vi "ZLIB Transfer Raw File__ogtk.vi"(5 "error in (no error)":errorcluster, 6 "compressed size":u32, 7 "unzip Refnum":T1, 8 "zip Refnum":T2) -> (0 "error out":errorcluster, 2 "unzip Refnum out":T1, 3 "zip Refnum out":T2)   [LabVIEW 2012]
doc: "Copies a file in raw mode from an unzip session into the ZIP file. Both file sessions must have been opened in raw mode, otherwise the created archive will be corrupted."
uses:
  <userlib>/_OpenG.lib/lvzip/lvzip.llb/ZLIB Unzip Handle__ogtk.ctl
  <userlib>/_OpenG.lib/lvzip/lvzip.llb/ZLIB Zip Handle__ogtk.ctl
  <userlib>/_OpenG.lib/lvzip/lvzlib.dll
panel:
  # "Please visit http://www.OpenG.org to learn about the\nOpen Source LabVIEW software movement.\n\nNOTICE -- YOU MUST LEAVE THIS NOTICE IN PLACE.  PER THE TERMS OF THE LICENSE BELOW, YOU MAY SUBLICENSE THIS SOFTWARE \nIN ANY WAY THAT DOES NOT CONFLICT WITH THIS LICENSE.\n\n### BSD License (http://www.opensource.org/licenses/bsd-license.php) Begin ###\n \nCopyright (C) 2002-2004 Rolf Kalbermatter rolf.kalbermatter@citeng.com\nCopyright (C) 2002 Jim Kring jim@jimkring.com\n\nAll rights reserved.\n\nRedistribution and use in source and binary forms, with or without modification, are permitted provided that the following conditions are met:\n\n    * Redistributions of source code must retain the above copyright notice, this list of conditions and the following disclaimer.\n    * Redistributions in binary form must reproduce the above copyright notice, this list of conditions and the following disclaimer in the \n       documentation and/or other materials provided with the distribution.\n    * Neither the name of SciWare, James Kring, Inc., nor the names of its contributors may be used to endorse or promote products derived \n       from this software without specific prior written permission.\n\nTHIS SOFTWARE IS PROVIDED BY THE COPYRIGHT HOLDERS AND CONTRIBUTORS \"AS IS\" AND ANY EXPRESS OR IMPLIED WARRANTIES, \nINCLUDING, BUT NOT LIMITED TO, THE IMPLIED WARRANTIES OF MERCHANTABILITY AND FITNESS FOR A PARTICULAR PURPOSE ARE \nDISCLAIMED. IN NO EVENT SHALL THE COPYRIGHT OWNER OR CONTRIBUTORS BE LIABLE FOR ANY DIRECT, INDIRECT, INCIDENTAL,\n SPECIAL, EXEMPLARY, OR CONSEQUENTIAL DAMAGES (INCLUDING, BUT NOT LIMITED TO, PROCUREMENT OF SUBSTITUTE GOODS OR \nSERVICES; LOSS OF USE, DATA, OR PROFITS; OR BUSINESS INTERRUPTION) HOWEVER CAUSED AND ON ANY THEORY OF LIABILITY, \nWHETHER IN CONTRACT, STRICT LIABILITY, OR TORT (INCLUDING NEGLIGENCE OR OTHERWISE) ARISING IN ANY WAY OUT OF THE USE \nOF THIS SOFTWARE, EVEN IF ADVISED OF THE POSSIBILITY OF SUCH DAMAGE.\n\n### BSD License End ###"
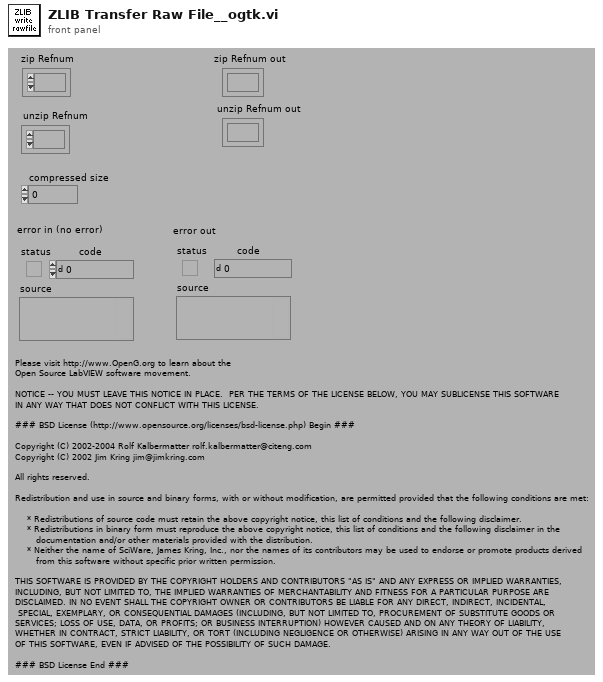
[diagram p1: front panel]
types:
  T1 = typedef "ZLIB Unzip Handle__ogtk.ctl" = refnum<k1>
  T2 = typedef "ZLIB Zip Handle__ogtk.ctl" = refnum<k1>
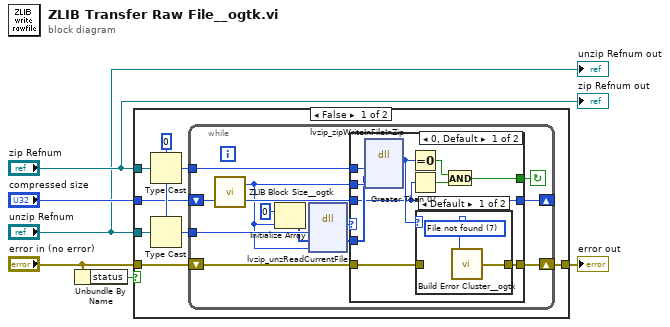
[diagram p0: block diagram]
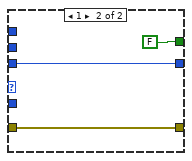
[diagram p3: hidden frame]
diagram:
  n1 = Unbundle By Name("error in (no error)") -> ("status"=w5:bool)
  n2 = case shown="False" w5 {
    tunnel: "error in (no error)" -> [w11 w44]
    tunnel: [w8 w44] -> w6
    tunnel: "zip Refnum" -> [w13 _]
    tunnel: "unzip Refnum" -> [w10 _]
    tunnel: "compressed size" -> [w7 _]
    frame False {
      w12 = u32 0 ("unzFile")
      n3 = Type Cast(type=w12, x=w13) -> (*(type *) &x=w14:u32)
      n4 = Type Cast(type=w12, x=w10) -> (*(type *) &x=w9:u32)
      n5 = while {
        tunnel: w9 -> [w19]
        shift-left: w7 -> [w24]
        shift-right: [w22] -> _
        shift-left: w11 -> [w15]
        shift-right: [w26] -> w8
        tunnel: w14 -> [w27]
        stop <- w25 continue-if-true
        n6 = call <userlib>:"ZLIB Block Size__ogtk.vi"("length in"=w24) -> ("length rem"=w23:u32, "block len"=w17:u32)  [unwired: 1 in]
        n7 = Initialize Array(u8 0 ("Element Data"), w17) -> (w16:u8[])
        n8 = dll-call lib="C:/Program Files/National Instruments/LabVIEW 2012/user.lib/_OpenG.lib/lvzip/lvzlib.*" fn="lvzip_unzReadCurrentFile"("unzFile"=w19, "buffer"=w16, "size"=w17) -> (w21:i32, "buffer"=w20:u8[])  [unwired: 5 in, 2 out]
        n9 = case shown="0, Default" w21 {
          tunnel: w27 -> [w37 _]
          tunnel: w17 -> [w36 _]
          tunnel: [w34 w42] -> w26
          tunnel: w20 -> [w33 _]
          tunnel: w15 -> [w32 w42]
          tunnel: [w29 FALSE] -> w25
          tunnel: w23 -> [w28 w41]
          tunnel: [w28 w41] -> w22
          frame 0, Default {
            n10 = dll-call lib="C:/Program Files/National Instruments/LabVIEW 2012/user.lib/_OpenG.lib/lvzip/lvzlib.*" fn="lvzip_zipWriteInFileInZip"("unzFile"=w37, "buffer"=w33, "size"=w36) -> (w35:i32)  [unwired: 6 in, 2 out]
            n11 = Equal To 0?(x=w35) -> (x = 0?=w31:bool)
            n12 = Greater Than 0?(x=w28) -> (x > 0?=w30:bool)
            n13 = case shown="Default" w35 {
              tunnel: w32 -> [_ w40]
              tunnel: [w39 w40] -> w34
              frame Default {
                w38 = 7 items=["No error", "Argument error", "Memory is full", "Out of zone", "End of file", "File already open", "Generic file I/O error", "File not found", "File permission error", "Disk is full", "Duplicate path", "Too many files open", "System feature not enabled", "Resource file not found", "Cannot add resource", "Resource not found", "Image not found", "Image memory error", "Pen does not exist", "Config type invalid", "Config token not found", "Config parse error", "Config memory error", "Bad external code format", "Bad external code offset", "External code not present", "Null window", "Destroy window error", "Null menu", "Print aborted", "Bad print record", "Print driver error", "Windows error during printing", "Memory error during printing", "Print dialog error", "Generic print error", "Invalid device refnum", "Device not found", "Device parameter error", "Device unit error", "Cannot open device", "Device call aborted", "Generic error", "Cancelled by user", "Object ID too low", "Object ID too high", "Object not in heap", "Unknown heap", "Unknown object (invalid DefProc)", "Unknown object (DefProc not in table)", "Message out of range", "Invalid (null) method", "Unknown message", "Manager call not supported", "Bad address", "Network operation in progress", "Network operation timed out", "Connection is busy", "Network attribute not supported", "Network error", "Address in use", "System out of memory", "Connection aborted", "Connection refused", "Not connected", "Already connected", "Connection closed", "Initialization error (interapplication manager)", "Bad occurrence", "Wait on unbound occurrence handler", "Occurrence queue overflow", "Datalog type conflict", "Unused", "Unrecognized type (interapplication manager)", "Memory corrupt", "Failed to make temporary DLL", "Old CIN version", "Drag socket not found", "Failed to load drop-object", "Failed to register OLE object", "Failed to release OLE object", "Format specifier type mismatch", "Unknown format specifier", "Too few format specifiers", "Too many format specifiers", "Scan failed", "Newer CIN version", "Error converting to variant", "Runtime menu error", "Password tampered", "Variant attribute not found", "Incompatible variant data type", "Event data is not available", "Event Store is not present", "Occurrence is not found", "Event Queue is not created", "Event info is not available", "Refnum passed is NULL", "Error retrieving Class GUID", "Error retrieving CoClass GUID", "Error retrieving TypeLib GUID.", "Bad built application magic bytes.", "Specific driver is different from the specific driver associated with the Logical Name.", "There is no session opened to the class driver.", "Max Error", "MAX - Error with config objects", "MAX - Error loading configuration", "MAX - Group not supported"]
                n14 = call <userlib>:"Build Error Cluster__ogtk.vi"("code"=w38) -> ("error out"=w39:errorcluster)  [unwired: 1 in]
              }
              frame 0 {
              }
            }
            n15 = And(x=w31, y=w30) -> (x .and. y?=w29:bool)
          }
          frame 1 {
          }
        }
      }
    }
    frame True {
    }
  }
  "error out" <- w6
  "zip Refnum out" <- "zip Refnum"
  "unzip Refnum out" <- "unzip Refnum"
